vi "DB Read Queries.vi"(5 "Query info":T2, 7 "Query Command":T1, 8 "에러 입력(에러 없음)":errorcluster, 11 "참조 번호 입력":T3) -> (0 "에러 출력":errorcluster, 1 "Data (0번행)":string[](array[string]), 2 "Data":string[][](array[string]), 3 "참조 번호 출력":T3, 4 "None?":bool)   [LabVIEW 2020]
uses:
  <vilib>/addons/database/Connection.llb/Conn ObjectReference.ctl
  Controls/Clst_Query Info.ctl
  Controls/Cmd_Read Query.ctl
  Variables/Global_Cal Info.vi
  <vilib>/addons/database/NI_Database_API.lvlib
panel:
  out "Query":string
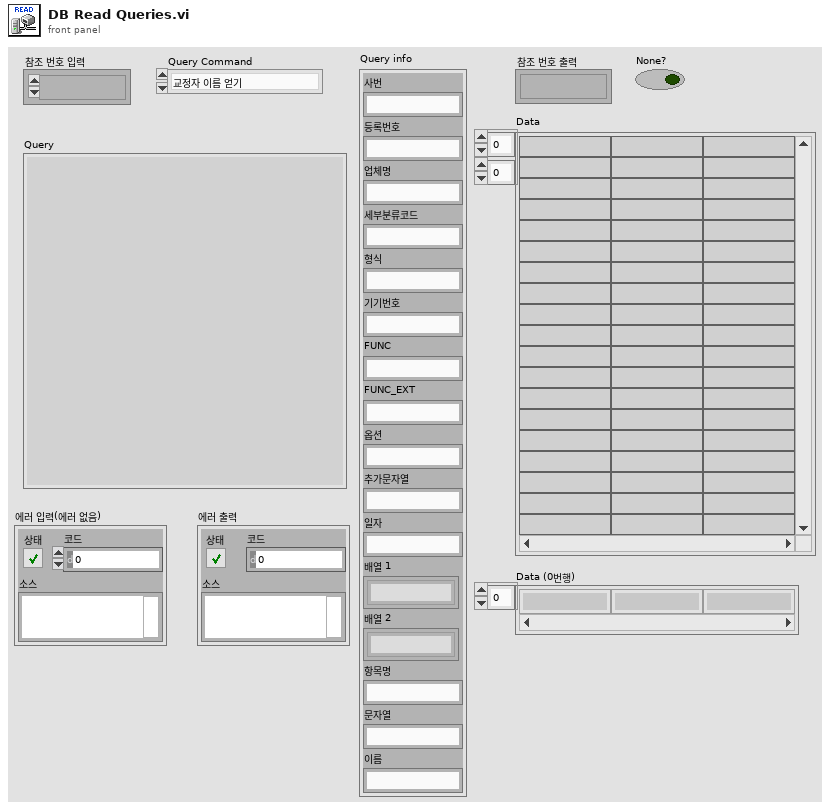
[diagram p1: front panel]
types:
  T1 = typedef "Cmd_Read Query.ctl" = enum16{"교정자 이름 얻기", "인증교정자 얻기", "기술책임자 얻기", "기책부책 얻기", "등록번호 얻기", "등록정보 얻기", "업체정보 얻기", "교정일자(CAMAS) 얻기", "교정일자(CALSTD) 얻기", "교정환경 얻기", "교정절차서 목록 얻기", "교정절차서명 얻기", "교정절차 목록얻기", "교정절차 얻기", "PROC 교정절차 얻기", "PROC SPEC 얻기", "교정절차(Func별) 얻기", "교정절차(Func_ext별) 얻기", "기관코드 얻기", "교정기능(세부분류) 얻기", "교정기능(모델) 얻기", "교정기능 목록 얻기", "교정기능 명칭 얻기", "교정기능 항목명칭 얻기", "DB (사용기준기) 얻기", "DB (기준기이름) 얻기", "DB (기준기이름목록) 얻기", "DB (기준기목록) 얻기", "DB (기준기값) 얻기", "DB (CMC) 얻기", "DB (FUNC) 얻기", "DB (CALNAME) 얻기", "DB (STDNAME) 얻기", "DB (SPEC) 얻기", "모델(항목전체) 얻기", "모델(최대범위) 얻기", "모델(최소범위) 얻기", "모델(최대최소) 얻기", "모델(범위조건) 얻기", "모델(등록요청) 얻기", "모델(형식별) 얻기", "모델(조건별) 얻기", "모델(모델검색) 얻기", "세부분류 목록 얻기", "기준기등록리스트 얻기", "STD Cal Date Check", "DB등록일자 얻기", "적용항목 얻기", "기타정보 얻기", "기준기요청 얻기", "서버버전 얻기"}
  T2 = typedef "Clst_Query Info.ctl" = cluster{"사번":string, "등록번호":string, "업체명":string, "세부분류코드":string, "형식":string, "기기번호":string, "FUNC":string, "FUNC_EXT":string, "옵션":string, "추가문자열":string, "일자":string, "배열 1":string[], "배열 2":string[], "항목명":string, "문자열":string, "이름":string}
  T3 = typedef "NI_Database_API.lvlib/Conn ObjectReference.ctl" = refnum<k1>
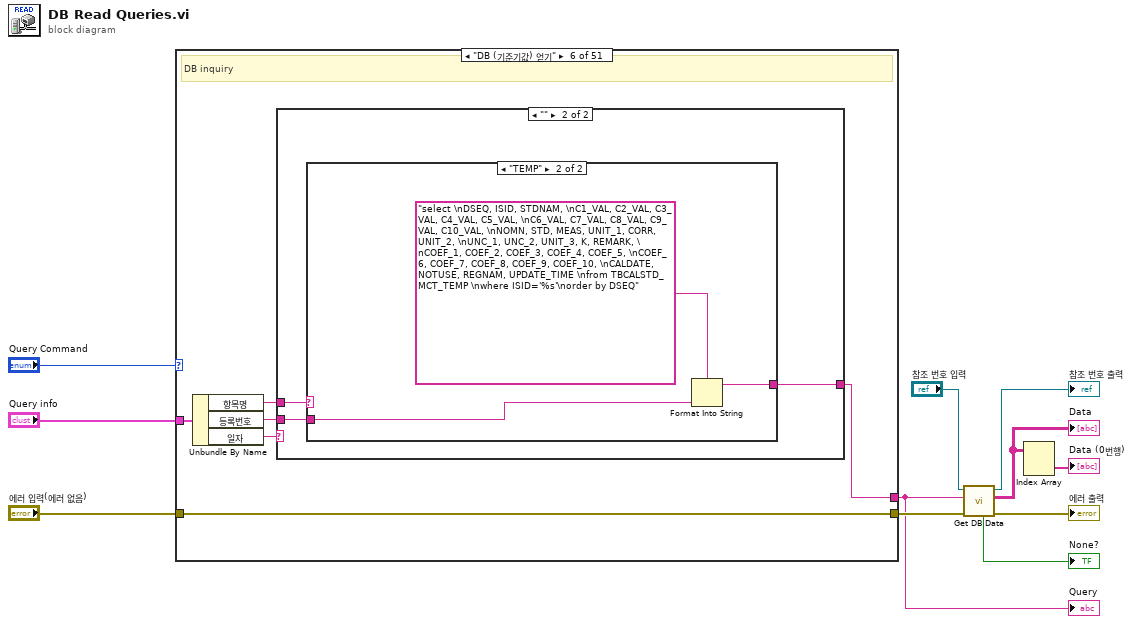
[diagram p0: block diagram]
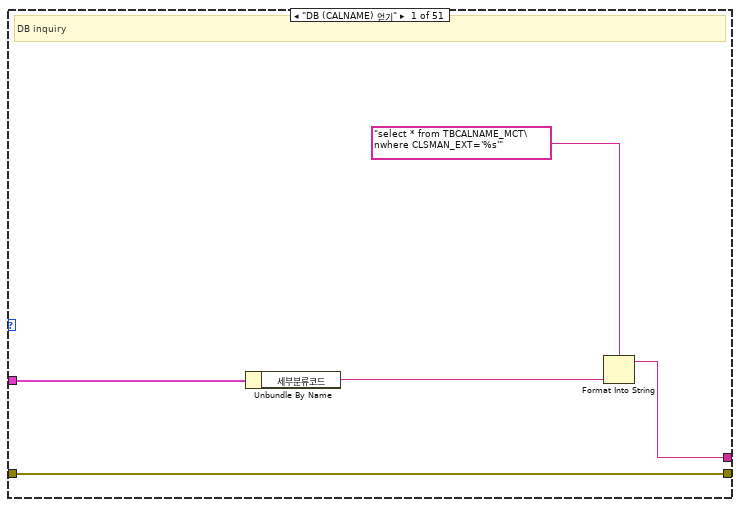
[diagram p2: hidden frame]
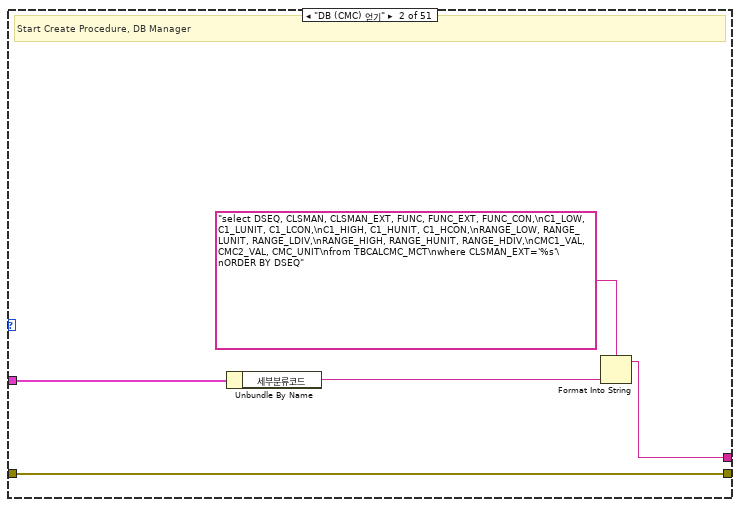
[diagram p3: hidden frame]
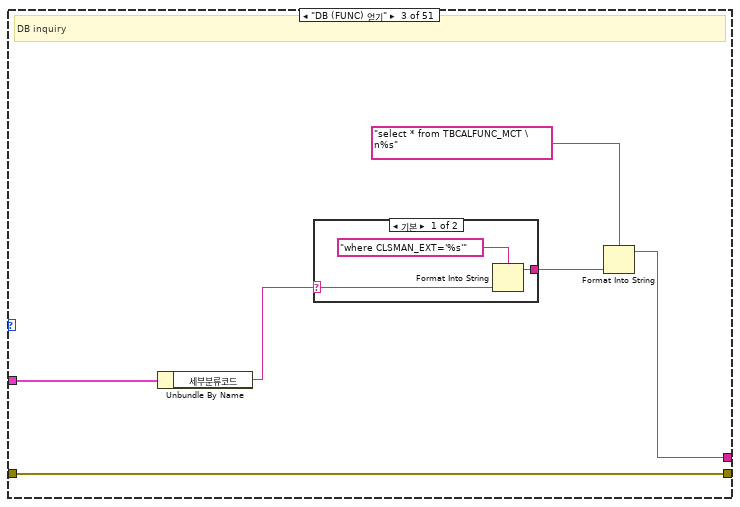
[diagram p4: hidden frame]
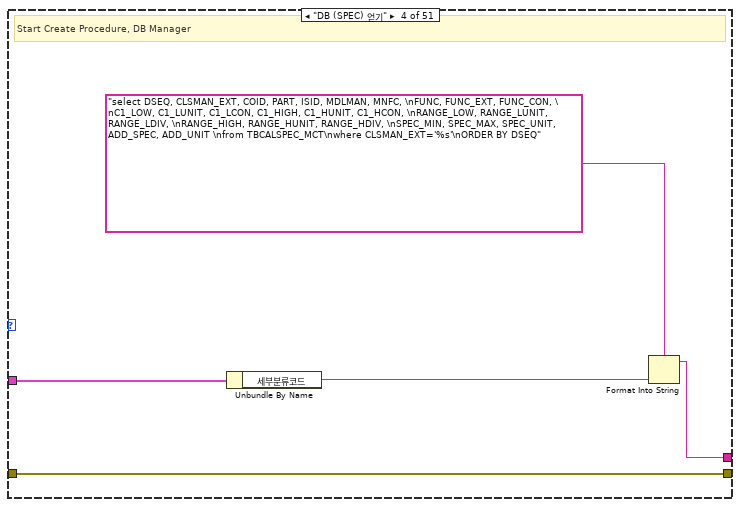
[diagram p6: hidden frame]
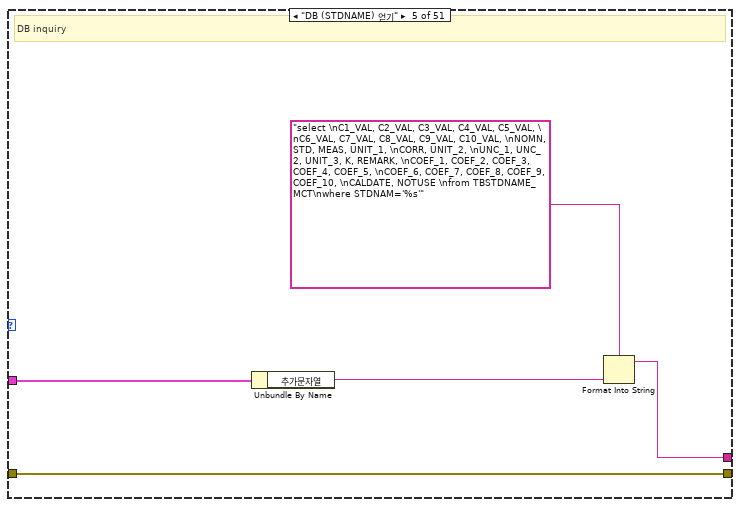
[diagram p7: hidden frame]
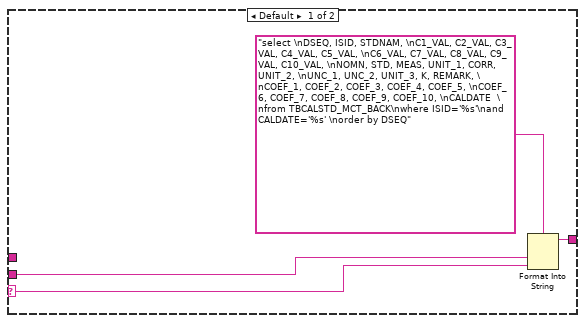
[diagram p8: hidden frame]
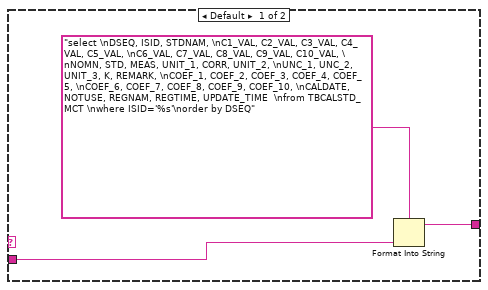
[diagram p9: hidden frame]
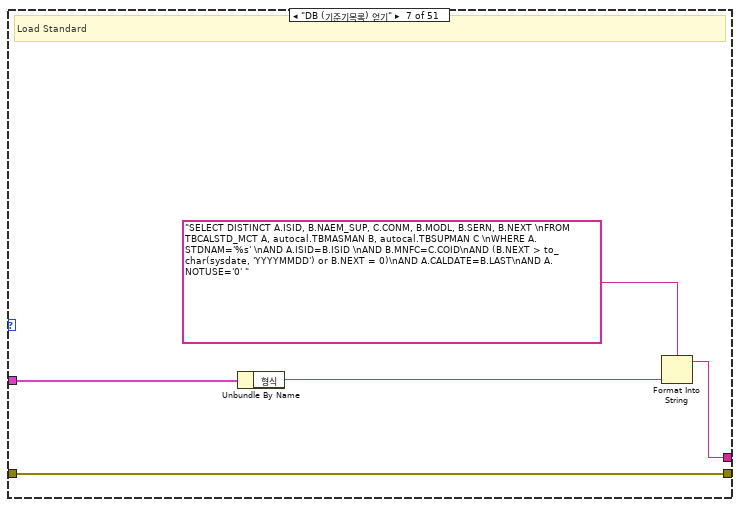
[diagram p10: hidden frame]
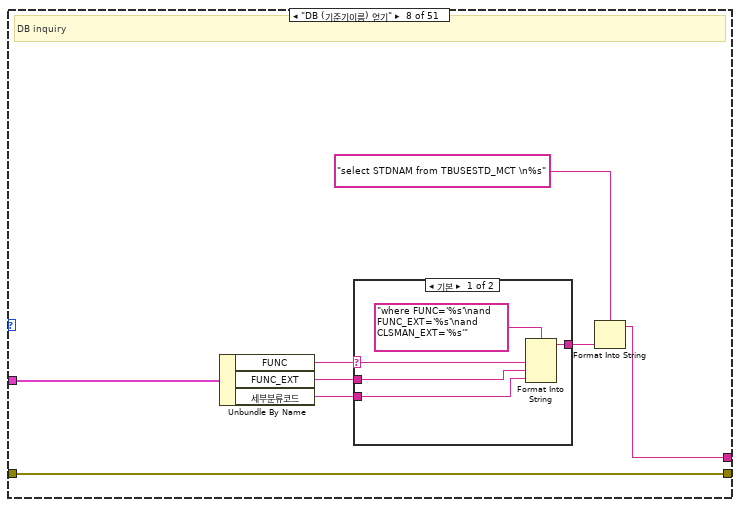
[diagram p11: hidden frame]
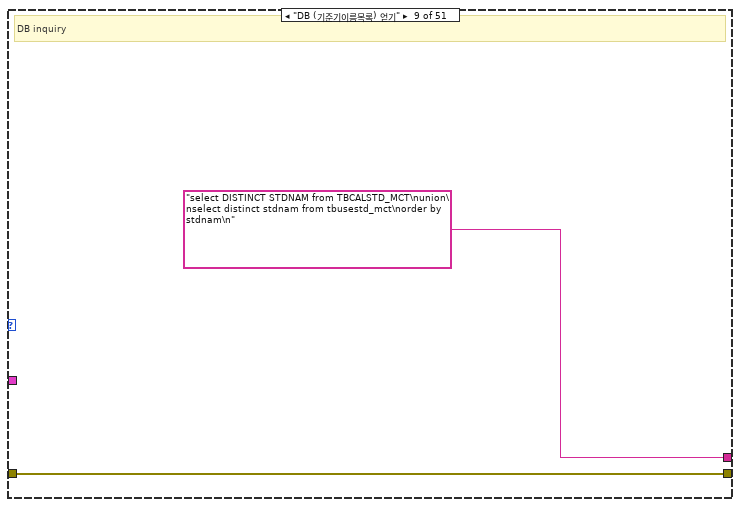
[diagram p13: hidden frame]
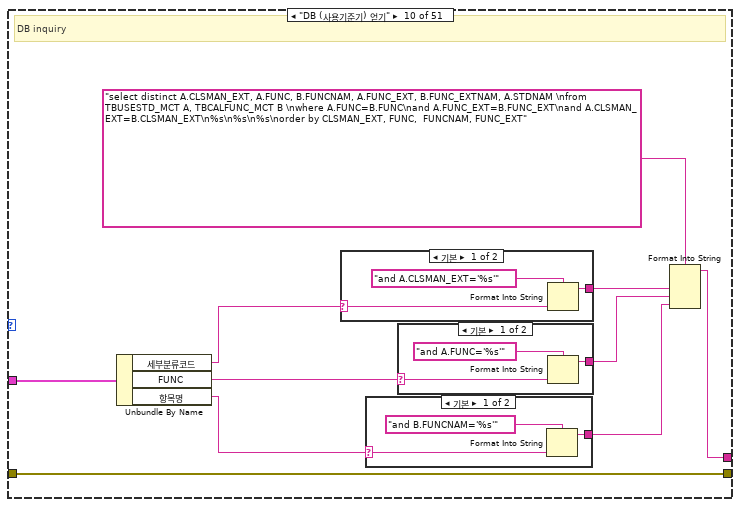
[diagram p14: hidden frame]
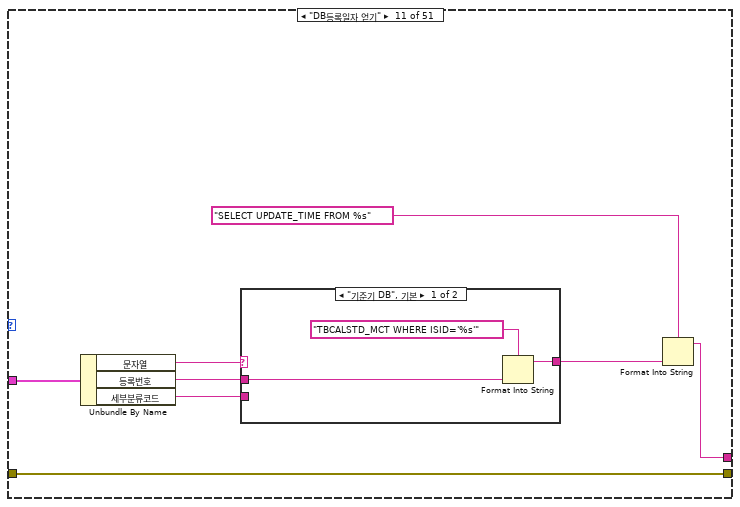
[diagram p18: hidden frame]
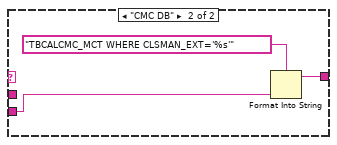
[diagram p19: hidden frame]
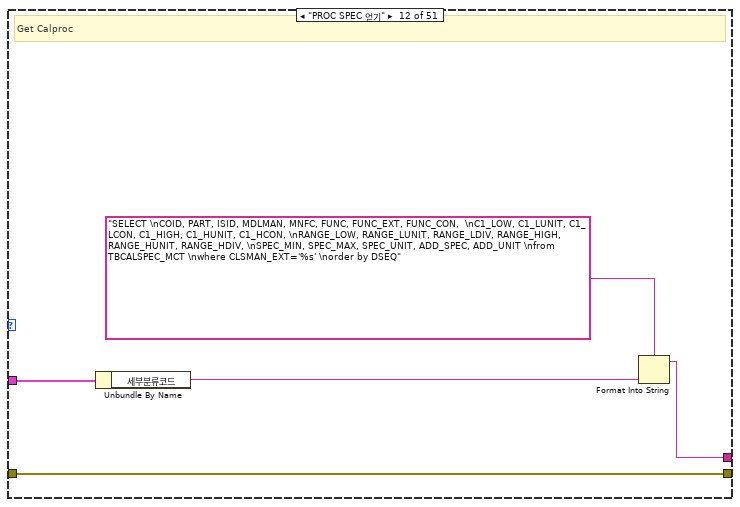
[diagram p20: hidden frame]
diagram:
  n1 = case shown="\"DB (기준기값) 얻기\"" "Query Command" {
    tunnel: "에러 입력(에러 없음)" -> [w16 w21 w27 w35 w40 w46 w64 w72 w79 w89 w106 w117 w127 w138 w155 w160 w165 w175 w186 w191 w196 w201 w209 w229 w248 w267 w278 w283 w304 w327 w332 w357 w365 w371 w376 w377 w386 w388 w397 w414 w431 w442 w457 w464 w476 w484 w490 w492 w497 w507 w521]
    tunnel: [w16 w21 w27 w35 w40 w46 w64 w72 w79 w89 w106 w117 w127 w138 w155 w160 w165 w175 w186 w191 w196 w201 w209 w229 w248 w267 w278 w283 w304 w327 w332 w357 w365 w371 w376 w377 w386 w388 w397 w414 w431 w442 w457 w464 w476 w484 w490 w492 w497 w507 w521] -> w6
    tunnel: "Query info" -> [w14 w20 w26 w34 w38 w45 w62 w71 _ w88 w105 w114 w118 w135 w154 _ w164 w174 w185 w190 w194 w197 w208 w226 w245 w264 w277 w282 w294 w326 w335 w353 w363 _ w375 w380 w384 _ w392 w413 w428 w441 w456 w463 w475 w483 _ _ w495 w506 _]
    tunnel: [w12 w17 w24 w31 w36 w42 w60 w69 "select DISTINCT STDNAM from TBCALSTD_MCT\nunion\nselect distinct stdnam from tbusestd_mct\norder by stdnam\n" w86 w103 w113 w123 w136 w152 "select CLSMAN_EXT, FUNC, FUNCNAM, FUNC_EXT, FUNC_EXTNAM\nfrom TBCALFUNC_MCT\norder by clsman_ext" ("포맷 문자열") w162 w172 w182 w188 w192 w200 w202 w228 w247 w266 w274 w279 w303 w323 w333 w354 w364 "select distinct emid from autocal.tbcetman\nwhere clas='기술책임자(정)'\nor clas='기술책임자(부)'\norder by emid" ("SQL query") w373 w378 w382 "SELECT DISTINCT REGTYP, CLSMAN_EXT, EQPNAM, MDLMAN, OPT_CODE, REGNAM, \nSUBSTR(UPDATE_TIME,0, 10) \nFROM TBCALPROC_MCT_TEMP \nORDER BY CLSMAN_EXT, MDLMAN, OPT_CODE" w393 w410 w429 w440 w455 w462 w472 w481 "SELECT mct_ver, ftp_ver FROM TBMCTVERMAN" ("SQL query") "select distinct clsman_ext, coddes_ext\nfrom autocal.tbclsman\nwhere stdnam is not null\norder by clsman_ext" ("SQL query") w493 w502 "SELECT DISTINCT A.CLSMAN_EXT, B.CODDES_EXT\nFROM\nTBCALFUNC_MCT A, AUTOCAL.TBCLSMAN B\nWHERE A.CLSMAN_EXT=B.CLSMAN_EXT\nORDER BY A.CLSMAN_EXT"] -> w3
    frame "DB (CALNAME) 얻기" {
      # "DB inquiry"
      n2 = Unbundle By Name(w14) -> ("세부분류코드"=w15:string)
      n3 = Format Into String(format string="select * from TBCALNAME_MCT\nwhere CLSMAN_EXT='%s'", w15) -> (resulting string=w12:string)  [unwired: 2 in, 1 out]
    }
    frame "DB (CMC) 얻기" {
      # "Start Create Procedure, DB Manager"
      n4 = Unbundle By Name(w20) -> ("세부분류코드"=w18:string)
      n5 = Format Into String(format string="select DSEQ, CLSMAN, CLSMAN_EXT, FUNC, FUNC_EXT, FUNC_CON,\nC1_LOW, C1_LUNIT, C1_LCON,\nC1_HIGH, C1_HUNIT, C1_HCON,\nRANGE_LOW, RANGE_LUNIT, RANGE_LDIV,\nRANGE_HIGH, RANGE_HUNIT, RANGE_HDIV,\nCMC1_VAL, CMC2_VAL, CMC_UNIT\nfrom TBCALCMC_MCT\nwhere CLSMAN_EXT='%s'\nORDER BY DSEQ", w18) -> (resulting string=w17:string)  [unwired: 2 in, 1 out]
    }
    frame "DB (FUNC) 얻기" {
      # "DB inquiry"
      n6 = Unbundle By Name(w26) -> ("세부분류코드"=w23:string)
      n7 = case shown="기본" w23 {
        selector: w23 -> [w30 _]
        tunnel: [w29 _] -> w22
        frame Default {
          n8 = Format Into String(format string="where CLSMAN_EXT='%s'", w30) -> (resulting string=w29:string)  [unwired: 2 in, 1 out]
        }
        frame "" {
        }
      }
      n9 = Format Into String(format string="select * from TBCALFUNC_MCT \n%s", w22) -> (resulting string=w24:string)  [unwired: 2 in, 1 out]
    }
    frame "DB (SPEC) 얻기" {
      # "Start Create Procedure, DB Manager"
      n10 = Unbundle By Name(w34) -> ("세부분류코드"=w32:string)
      n11 = Format Into String(format string="select DSEQ, CLSMAN_EXT, COID, PART, ISID, MDLMAN, MNFC, \nFUNC, FUNC_EXT, FUNC_CON, \nC1_LOW, C1_LUNIT, C1_LCON, C1_HIGH, C1_HUNIT, C1_HCON, \nRANGE_LOW, RANGE_LUNIT, RANGE_LDIV, \nRANGE_HIGH, RANGE_HUNIT, RANGE_HDIV, \nSPEC_MIN, SPEC_MAX, SPEC_UNIT, ADD_SPEC, ADD_UNIT \nfrom TBCALSPEC_MCT\nwhere CLSMAN_EXT='%s'\nORDER BY DSEQ", w32) -> (resulting string=w31:string)  [unwired: 2 in, 1 out]
    }
    frame "DB (STDNAME) 얻기" {
      # "DB inquiry"
      n12 = Unbundle By Name(w38) -> ("추가문자열"=w39:string)
      n13 = Format Into String(format string="select \nC1_VAL, C2_VAL, C3_VAL, C4_VAL, C5_VAL, \nC6_VAL, C7_VAL, C8_VAL, C9_VAL, C10_VAL, \nNOMN, STD, MEAS, UNIT_1, \nCORR, UNIT_2, \nUNC_1, UNC_2, UNIT_3, K, REMARK, \nCOEF_1, COEF_2, COEF_3, COEF_4, COEF_5, \nCOEF_6, COEF_7, COEF_8, COEF_9, COEF_10, \nCALDATE, NOTUSE \nfrom TBSTDNAME_MCT\nwhere STDNAM='%s'", w39) -> (resulting string=w36:string)  [unwired: 2 in, 1 out]
    }
    frame "DB (기준기값) 얻기" {
      # "DB inquiry"
      n14 = Unbundle By Name(w45) -> ("항목명"=w41:string, "등록번호"=w43:string, "일자"=w44:string)
      n15 = case shown="\"\"" w44 {
        selector: w44 -> [w50 _]
        tunnel: w43 -> [w49 w53]
        tunnel: [w47 w52] -> w42
        tunnel: w41 -> [_ w51]
        frame Default {
          n16 = Format Into String(format string="select \nDSEQ, ISID, STDNAM, \nC1_VAL, C2_VAL, C3_VAL, C4_VAL, C5_VAL, \nC6_VAL, C7_VAL, C8_VAL, C9_VAL, C10_VAL, \nNOMN, STD, MEAS, UNIT_1, CORR, UNIT_2, \nUNC_1, UNC_2, UNIT_3, K, REMARK, \nCOEF_1, COEF_2, COEF_3, COEF_4, COEF_5, \nCOEF_6, COEF_7, COEF_8, COEF_9, COEF_10, \nCALDATE  \nfrom TBCALSTD_MCT_BACK\nwhere ISID='%s'\nand CALDATE='%s' \norder by DSEQ", w49, w50) -> (resulting string=w47:string)  [unwired: 2 in, 1 out]
        }
        frame "" {
          n17 = case shown="\"TEMP\"" w51 {
            tunnel: w53 -> [w55 w58]
            tunnel: [w54 w57] -> w52
            frame Default {
              n18 = Format Into String(format string="select \nDSEQ, ISID, STDNAM, \nC1_VAL, C2_VAL, C3_VAL, C4_VAL, C5_VAL, \nC6_VAL, C7_VAL, C8_VAL, C9_VAL, C10_VAL, \nNOMN, STD, MEAS, UNIT_1, CORR, UNIT_2, \nUNC_1, UNC_2, UNIT_3, K, REMARK, \nCOEF_1, COEF_2, COEF_3, COEF_4, COEF_5, \nCOEF_6, COEF_7, COEF_8, COEF_9, COEF_10, \nCALDATE, NOTUSE, REGNAM, REGTIME, UPDATE_TIME  \nfrom TBCALSTD_MCT \nwhere ISID='%s'\norder by DSEQ", w55) -> (resulting string=w54:string)  [unwired: 2 in, 1 out]
            }
            frame "TEMP" {
              n19 = Format Into String(format string="select \nDSEQ, ISID, STDNAM, \nC1_VAL, C2_VAL, C3_VAL, C4_VAL, C5_VAL, \nC6_VAL, C7_VAL, C8_VAL, C9_VAL, C10_VAL, \nNOMN, STD, MEAS, UNIT_1, CORR, UNIT_2, \nUNC_1, UNC_2, UNIT_3, K, REMARK, \nCOEF_1, COEF_2, COEF_3, COEF_4, COEF_5, \nCOEF_6, COEF_7, COEF_8, COEF_9, COEF_10, \nCALDATE, NOTUSE, REGNAM, UPDATE_TIME \nfrom TBCALSTD_MCT_TEMP \nwhere ISID='%s'\norder by DSEQ", w58) -> (resulting string=w57:string)  [unwired: 2 in, 1 out]
            }
          }
        }
      }
    }
    frame "DB (기준기목록) 얻기" {
      # "Load Standard"
      n20 = Unbundle By Name(w62) -> ("형식"=w61:string)
      n21 = Format Into String(format string="SELECT DISTINCT A.ISID, B.NAEM_SUP, C.CONM, B.MODL, B.SERN, B.NEXT \nFROM TBCALSTD_MCT A, autocal.TBMASMAN B, autocal.TBSUPMAN C \nWHERE A.STDNAM='%s' \nAND A.ISID=B.ISID \nAND B.MNFC=C.COID\nAND (B.NEXT > to_char(sysdate, 'YYYYMMDD') or B.NEXT = 0)\nAND A.CALDATE=B.LAST\nAND A.NOTUSE='0' ", w61) -> (resulting string=w60:string)  [unwired: 2 in, 1 out]
    }
    frame "DB (기준기이름) 얻기" {
      # "DB inquiry"
      n22 = Unbundle By Name(w71) -> ("FUNC"=w66:string, "FUNC_EXT"=w68:string, "세부분류코드"=w65:string)
      n23 = case shown="기본" w66 {
        selector: w66 -> [w74 _]
        tunnel: w68 -> [w76 _]
        tunnel: [w75 _] -> w67
        tunnel: w65 -> [w73 _]
        frame Default {
          n24 = Format Into String(format string="where FUNC='%s'\nand FUNC_EXT='%s'\nand CLSMAN_EXT='%s'" ("포맷 문자열"), w74, w76, w73) -> (resulting string=w75:string)  [unwired: 2 in, 1 out]
        }
        frame "" {
        }
      }
      n25 = Format Into String(format string="select STDNAM from TBUSESTD_MCT \n%s", w67) -> (resulting string=w69:string)  [unwired: 2 in, 1 out]
    }
    frame "DB (기준기이름목록) 얻기" {
      # "DB inquiry"
    }
    frame "DB (사용기준기) 얻기" {
      # "DB inquiry"
      n26 = Unbundle By Name(w88) -> ("세부분류코드"=w81:string, "FUNC"=w85:string, "항목명"=w83:string)
      n27 = case shown="기본" w81 {
        selector: w81 -> [w92 _]
        tunnel: [w91 _] -> w80
        frame Default {
          n28 = Format Into String(format string="and A.CLSMAN_EXT='%s'" ("포맷 문자열"), w92) -> (resulting string=w91:string)  [unwired: 2 in, 1 out]
        }
        frame "" {
        }
      }
      n29 = case shown="기본" w83 {
        selector: w83 -> [w95 _]
        tunnel: [w94 _] -> w82
        frame Default {
          n30 = Format Into String(format string="and B.FUNCNAM='%s'" ("포맷 문자열"), w95) -> (resulting string=w94:string)  [unwired: 2 in, 1 out]
        }
        frame "" {
        }
      }
      n31 = case shown="기본" w85 {
        selector: w85 -> [w98 _]
        tunnel: [w97 _] -> w84
        frame Default {
          n32 = Format Into String(format string="and A.FUNC='%s'" ("포맷 문자열"), w98) -> (resulting string=w97:string)  [unwired: 2 in, 1 out]
        }
        frame "" {
        }
      }
      n33 = Format Into String(format string="select distinct A.CLSMAN_EXT, A.FUNC, B.FUNCNAM, A.FUNC_EXT, B.FUNC_EXTNAM, A.STDNAM \nfrom TBUSESTD_MCT A, TBCALFUNC_MCT B \nwhere A.FUNC=B.FUNC\nand A.FUNC_EXT=B.FUNC_EXT\nand A.CLSMAN_EXT=B.CLSMAN_EXT\n%s\n%s\n%s\norder by CLSMAN_EXT, FUNC,  FUNCNAM, FUNC_EXT", w80, w84, w82) -> (resulting string=w86:string)  [unwired: 2 in, 1 out]
    }
    frame "DB등록일자 얻기" {
      n34 = Unbundle By Name(w105) -> ("문자열"=w102:string, "등록번호"=w100:string, "세부분류코드"=w99:string)
      n35 = case shown="\"기준기 DB\", 기본" w102 {
        tunnel: [w107 w111] -> w101
        tunnel: w100 -> [w108 _]
        tunnel: w99 -> [_ w110]
        frame "기준기 DB", Default {
          n36 = Format Into String(format string="TBCALSTD_MCT WHERE ISID='%s'" ("포맷 문자열"), w108) -> (resulting string=w107:string)  [unwired: 2 in, 1 out]
        }
        frame "CMC DB" {
          n37 = Format Into String(format string="TBCALCMC_MCT WHERE CLSMAN_EXT='%s'" ("포맷 문자열"), w110) -> (resulting string=w111:string)  [unwired: 2 in, 1 out]
        }
      }
      n38 = Format Into String(format string="SELECT UPDATE_TIME FROM %s", w101) -> (resulting string=w103:string)  [unwired: 2 in, 1 out]
    }
    frame "PROC SPEC 얻기" {
      # "Get Calproc"
      n39 = Unbundle By Name(w114) -> ("세부분류코드"=w116:string)
      n40 = Format Into String(format string="SELECT \nCOID, PART, ISID, MDLMAN, MNFC, FUNC, FUNC_EXT, FUNC_CON,  \nC1_LOW, C1_LUNIT, C1_LCON, C1_HIGH, C1_HUNIT, C1_HCON, \nRANGE_LOW, RANGE_LUNIT, RANGE_LDIV, RANGE_HIGH, RANGE_HUNIT, RANGE_HDIV, \nSPEC_MIN, SPEC_MAX, SPEC_UNIT, ADD_SPEC, ADD_UNIT \nfrom TBCALSPEC_MCT \nwhere CLSMAN_EXT='%s' \norder by DSEQ", w116) -> (resulting string=w113:string)  [unwired: 2 in, 1 out]
    }
    frame "PROC 교정절차 얻기" {
      # "Get Calproc"
      n41 = Unbundle By Name(w118) -> ("추가문자열"=w122:string, "세부분류코드"=w125:string, "형식"=w126:string, "옵션"=w120:string)
      n42 = case shown="기본" w122 {
        tunnel: ["TBCALPROC_MCT" ("추가문자열") "TBCALPROC_MCT_TEMP" ("추가문자열")] -> w121
        frame Default {
        }
        frame "TEMP" {
        }
      }
      n43 = case shown="기본" w120 {
        selector: w120 -> [w129 _]
        tunnel: [w128 "AND OPT_CODE is null"] -> w119
        frame Default {
          n44 = Format Into String(format string="AND OPT_CODE='%s'", w129) -> (resulting string=w128:string)  [unwired: 2 in, 1 out]
        }
        frame "" {
        }
      }
      n45 = Format Into String(format string="SELECT\nDSEQ, FUNC, FUNC_EXT, \nCAL_VAL, CAL_UNIT, DISP_SYS, RESOL, RESOL_UNIT, \nC1_VAL, C2_VAL, C3_VAL, C4_VAL, C5_VAL,\nC6_VAL, C7_VAL, C8_VAL, C9_VAL, C10_VAL\nFROM %s\nWHERE CLSMAN_EXT='%s'\nAND MDLMAN='%s'\n%s\norder by DSEQ", w121, w125, w126, w119) -> (resulting string=w123:string)  [unwired: 2 in, 1 out]
    }
    frame "STD Cal Date Check" {
      n46 = Unbundle By Name(w135) -> ("옵션"=w134:string)
      n47 = case shown="\"2\"" w134 {
        tunnel: "select DISTINCT\nA.isid, B.naem_sup, TRIM(C.conm),\nB.modl, B.last, A.caldate, B.next,\nD.desn, E.desn\nfrom\nTBCALSTD_MCT A,\nautocal.TBMASMAN B,\nautocal.TBSUPMAN C,\nautocal.TBSTAMAN D, \nautocal.TBTYPMAN E\nwhere A.isid=B.isid \nAND B.mnfc=C.coid\nAND B.stat=D.stat\nAND B.tyep=E.tyep\nAND A.notuse='0'\n%s\norder by naem_sup" ("SQL query") -> [w139 w147]
        tunnel: [w140 w142] -> w136
        frame "1", Default {
          n48 = Format Into String(format string=w139, "AND A.caldate<>B.last" ("SQL query")) -> (resulting string=w140:string)  [unwired: 2 in, 1 out]
        }
        frame "2" {
          n49 = Format Date/Time String(time format string (%c)="%Y%m%d" ("시간 포맷 문자열 (%c)")) -> (date/time string=w145:string)  [unwired: 2 in]
          n50 = Format Into String(format string="AND B.next<'%s'\nAND B.next<>'0'" ("SQL query"), w145) -> (resulting string=w146:string)  [unwired: 2 in, 1 out]
          n51 = Format Into String(format string=w147, w146) -> (resulting string=w142:string)  [unwired: 2 in, 1 out]
        }
      }
    }
    frame "교정기능 명칭 얻기" {
      # "Get Cal Func List"
      n52 = Unbundle By Name(w154) -> ("FUNC"=w149:string, "세부분류코드"=w148:string, "FUNC_EXT"=w151:string)
      n53 = case shown="기본" w151 {
        selector: w151 -> [w157 _]
        tunnel: [w156 _] -> w150
        frame Default {
          n54 = Format Into String(format string="AND FUNC_EXT='%s'", w157) -> (resulting string=w156:string)  [unwired: 2 in, 1 out]
        }
        frame "" {
        }
      }
      n55 = Format Into String(format string="SELECT distinct func, funcnam, func_ext, func_extnam \nFROM TBCALFUNC_MCT \nWHERE FUNC='%s'\n%s\nAND CLSMAN_EXT='%s'", w149, w150, w148) -> (resulting string=w152:string)  [unwired: 2 in, 1 out]
    }
    frame "교정기능 목록 얻기" {
    }
    frame "교정기능 항목명칭 얻기" {
      # "DB Manager"
      n56 = Unbundle By Name(w164) -> ("세부분류코드"=w163:string)
      n57 = Format Into String(format string="select \nfunc, func_ext, \nc1_name, c2_name, c3_name, c4_name, c5_name, \nc6_name, c7_name, c8_name, c9_name, c10_name, \ncal_name, cal_unit, disp_sys, resol, resol_unit\nfrom TBCALNAME_MCT \nwhere \nCLSMAN_EXT='%s'" ("포맷 문자열"), w163) -> (resulting string=w162:string)  [unwired: 2 in, 1 out]
    }
    frame "교정기능(모델) 얻기" {
      # "Get Cal Func"
      n58 = Unbundle By Name(w174) -> ("추가문자열"=w168:string, "세부분류코드"=w173:string, "형식"=w170:string, "옵션"=w167:string)
      n59 = case shown="기본" w168 {
        tunnel: ["TBCALPROC_MCT" ("추가문자열") "TBCALPROC_MCT_TEMP" ("추가문자열")] -> w169
        frame Default {
        }
        frame "TEMP" {
        }
      }
      n60 = case shown="기본" w167 {
        selector: w167 -> [w177 _]
        tunnel: [w176 "AND OPT_CODE is null"] -> w166
        frame Default {
          n61 = Format Into String(format string="AND OPT_CODE='%s'", w177) -> (resulting string=w176:string)  [unwired: 2 in, 1 out]
        }
        frame "" {
        }
      }
      n62 = Format Into String(format string="select dseq, func, func_ext \nfrom %s\nwhere clsman_ext='%s' \nand mdlman='%s'\n%s\nORDER BY dseq", w169, w173, w170, w166) -> (resulting string=w172:string)  [unwired: 2 in, 1 out]
    }
    frame "교정기능(세부분류) 얻기" {
      # "Start Create Procedure"
      n63 = Unbundle By Name(w185) -> ("세부분류코드"=w183:string)
      n64 = Format Into String(format string="select A.func, A.funcnam, A.func_ext, A.func_extnam, B.coddes_ext\nfrom TBCALFUNC_MCT A, autocal.tbclsman B\nwhere A.clsman_ext='%s'\nAND A.clsman_ext=B.clsman_ext\norder by func_ext", w183) -> (resulting string=w182:string)  [unwired: 2 in, 1 out]
    }
    frame "교정일자(CALSTD) 얻기" {
      # "DB Manager"
      n65 = Unbundle By Name(w190) -> ("등록번호"=w189:string)
      n66 = Format Into String(format string="select distinct CALDATE \nfrom TBCALSTD_MCT_BACK \nwhere ISID='%s'\norder by CALDATE" ("SQL query"), w189) -> (resulting string=w188:string)  [unwired: 2 in, 1 out]
    }
    frame "교정일자(CAMAS) 얻기" {
      # "DB Manager"
      n67 = Unbundle By Name(w194) -> ("등록번호"=w193:string)
      n68 = Format Into String(format string="select LAST \nfrom autocal.tbmasman \nwhere ISID='%s'" ("SQL query"), w193) -> (resulting string=w192:string)  [unwired: 2 in, 1 out]
    }
    frame "교정자 이름 얻기", Default {
      # "Main, Get Basic Info"
      n69 = Unbundle By Name(w197) -> ("사번"=w198:string)
      n70 = Format Into String(format string="select emnm \nfrom autocal.tbempman \nwhere emid='%s' " ("포맷 문자열"), w198) -> (resulting string=w200:string)  [unwired: 2 in, 1 out]
    }
    frame "교정절차 목록얻기" {
      # "Get Cal Proc List"
      n71 = Unbundle By Name(w208) -> ("추가문자열"=w207:string, "세부분류코드"=w204:string, "형식"=w203:string)
      n72 = To Upper Case(1:w207) -> (0:w206:string)
      n73 = call <vilib>:"Trim Whitespace.vi"("string"=w206) -> ("trimmed string"=w205:string)  [unwired: 1 in]
      n74 = case shown="기본" w205 {
        tunnel: [w212 w216] -> w202
        tunnel: w204 -> [w210 w215]
        tunnel: w203 -> [w211 w214]
        frame Default {
          n75 = Format Into String(format string="select DISTINCT\nclsman, clsman_ext, eqpnam, mdlman, opt_code, c1_val\nfrom TBCALPROC_MCT\nwhere CLSMAN_EXT='%s'\nAND MDLMAN='설정'\nUNION\nselect DISTINCT\nclsman, clsman_ext, eqpnam, mdlman, opt_code, c1_val \nfrom TBCALPROC_MCT\nwhere CLSMAN_EXT='%s' \nAND MDLMAN='%s' \nUNION\nselect DISTINCT\nclsman, clsman_ext, eqpnam, mdlman, opt_code, c1_val \nfrom TBCALPROC_MCT\nwhere CLSMAN_EXT='%s' \nAND MDLMAN='ALL' \n\norder by mdlman, opt_code", w210, w210, w211, w210) -> (resulting string=w212:string)  [unwired: 2 in, 1 out]
        }
        frame "TEMP" {
          n76 = Format Into String(format string="select DISTINCT\nclsman, clsman_ext, eqpnam, mdlman, opt_code, c1_val \nfrom TBCALPROC_MCT_TEMP\nwhere CLSMAN_EXT='%s' \nAND MDLMAN='%s' \norder by mdlman, opt_code", w215, w214) -> (resulting string=w216:string)  [unwired: 2 in, 1 out]
        }
      }
    }
    frame "교정절차 얻기" {
      # "Insert proc_temp, DB Manager, DB inquiry"
      n77 = Unbundle By Name(w226) -> ("추가문자열"=w223:string, "세부분류코드"=w225:string, "형식"=w224:string, "옵션"=w219:string)
      n78 = To Upper Case(1:w223) -> (0:w222:string)
      n79 = call <vilib>:"Trim Whitespace.vi"("string"=w222) -> ("trimmed string"=w221:string)  [unwired: 1 in]
      n80 = case shown="기본" w219 {
        selector: w219 -> [w231 _]
        tunnel: [w230 "AND OPT_CODE is null"] -> w218
        frame Default {
          n81 = Format Into String(format string="AND OPT_CODE='%s'", w231) -> (resulting string=w230:string)  [unwired: 2 in, 1 out]
        }
        frame "" {
        }
      }
      n82 = case shown="기본" w221 {
        tunnel: ["TBCALPROC_MCT" ("추가문자열") "TBCALPROC_MCT_TEMP" ("추가문자열")] -> w220
        frame Default {
        }
        frame "TEMP" {
        }
      }
      n83 = Format Into String(format string="select \nDSEQ, CLSMAN, CLSMAN_EXT, EQPNAM, \nMDLMAN, OPT_CODE, FUNC, FUNC_EXT, \nC1_VAL, C2_VAL, C3_VAL, C4_VAL, C5_VAL, \nC6_VAL, C7_VAL, C8_VAL, C9_VAL, C10_VAL,\nCAL_VAL, CAL_UNIT, DISP_SYS, RESOL, RESOL_UNIT, \nREGNAM, UPDATE_TIME \nfrom %s\nwhere CLSMAN_EXT='%s' \nAND MDLMAN='%s'\n%s\norder by DSEQ", w220, w225, w224, w218) -> (resulting string=w228:string)  [unwired: 2 in, 1 out]
    }
    frame "교정절차(Func_ext별) 얻기" {
      # "Insert proc_temp, DB Manager, DB inquiry"
      n84 = Unbundle By Name(w245) -> ("추가문자열"=w242:string, "세부분류코드"=w244:string, "형식"=w243:string, "옵션"=w237:string, "FUNC"=w240:string)
      n85 = To Upper Case(1:w242) -> (0:w241:string)
      n86 = call <vilib>:"Trim Whitespace.vi"("string"=w241) -> ("trimmed string"=w239:string)  [unwired: 1 in]
      n87 = case shown="\"\"" w237 {
        selector: w237 -> [w250 _]
        tunnel: [w249 "AND OPT_CODE is null"] -> w236
        frame Default {
          n88 = Format Into String(format string="AND OPT_CODE='%s'", w250) -> (resulting string=w249:string)  [unwired: 2 in, 1 out]
        }
        frame "" {
        }
      }
      n89 = case shown="기본" w239 {
        tunnel: ["TBCALPROC_MCT" ("추가문자열") "TBCALPROC_MCT_TEMP" ("추가문자열")] -> w238
        frame Default {
        }
        frame "TEMP" {
        }
      }
      n90 = Format Into String(format string="select \nDSEQ, CLSMAN, CLSMAN_EXT, EQPNAM, \nMDLMAN, OPT_CODE, FUNC, FUNC_EXT,\nC1_VAL, C2_VAL, C3_VAL, C4_VAL, C5_VAL, \nC6_VAL, C7_VAL, C8_VAL, C9_VAL, C10_VAL,\nCAL_VAL, CAL_UNIT, DISP_SYS, RESOL, RESOL_UNIT\nfrom %s\nwhere CLSMAN_EXT='%s' \nAND MDLMAN='%s'\n%s\nAND FUNC_EXT='%s'\norder by DSEQ", w238, w244, w243, w236, w240) -> (resulting string=w247:string)  [unwired: 2 in, 1 out]
    }
    frame "교정절차(Func별) 얻기" {
      # "Insert proc_temp, DB Manager, DB inquiry"
      n91 = Unbundle By Name(w264) -> ("추가문자열"=w261:string, "세부분류코드"=w263:string, "형식"=w262:string, "옵션"=w256:string, "FUNC"=w259:string)
      n92 = To Upper Case(1:w261) -> (0:w260:string)
      n93 = call <vilib>:"Trim Whitespace.vi"("string"=w260) -> ("trimmed string"=w258:string)  [unwired: 1 in]
      n94 = case shown="\"\"" w256 {
        selector: w256 -> [w269 _]
        tunnel: [w268 "AND OPT_CODE is null"] -> w255
        frame Default {
          n95 = Format Into String(format string="AND OPT_CODE='%s'", w269) -> (resulting string=w268:string)  [unwired: 2 in, 1 out]
        }
        frame "" {
        }
      }
      n96 = case shown="기본" w258 {
        tunnel: ["TBCALPROC_MCT" ("추가문자열") "TBCALPROC_MCT_TEMP" ("추가문자열")] -> w257
        frame Default {
        }
        frame "TEMP" {
        }
      }
      n97 = Format Into String(format string="select \nDSEQ, CLSMAN, CLSMAN_EXT, EQPNAM, \nMDLMAN, OPT_CODE, FUNC, FUNC_EXT,\nC1_VAL, C2_VAL, C3_VAL, C4_VAL, C5_VAL, \nC6_VAL, C7_VAL, C8_VAL, C9_VAL, C10_VAL,\nCAL_VAL, CAL_UNIT, DISP_SYS, RESOL, RESOL_UNIT\nfrom %s\nwhere CLSMAN_EXT='%s' \nAND MDLMAN='%s'\n%s\nAND FUNC='%s'\norder by DSEQ", w257, w263, w262, w255, w259) -> (resulting string=w266:string)  [unwired: 2 in, 1 out]
    }
    frame "교정절차서 목록 얻기" {
      # "Get Cal Proc Docu List"
      n98 = Unbundle By Name(w277) -> ("사번"=w275:string)
      n99 = Format Into String(format string="select distinct A.stdnam, A.calstd, A.clsman \nfrom autocal.tbclsman A, autocal.tbcetman B \nwhere A.calcls=B.calcls \nand A.stdnam is not null \nand B.emid='%s' \nand B.clas='기술책임자(정)' \nand not (A.clsman='10615' or A.clsman='10622') \norder by A.clsman", w275) -> (resulting string=w274:string)  [unwired: 2 in, 1 out]
    }
    frame "교정절차서명 얻기" {
      # "Get Basic Info"
      n100 = Unbundle By Name(w282) -> ("세부분류코드"=w280:string)
      n101 = Format Into String(format string="select coddes, calstd \nfrom autocal.tbclsman \nwhere clsman_ext='%s'", w280) -> (resulting string=w279:string)  [unwired: 2 in, 1 out]
    }
    frame "교정환경 얻기" {
      # "Get Environment"
      n102 = Unbundle By Name(w294) -> ("세부분류코드"=w300:string, "일자"=w291:string)
      n103 = global read "Global_Cal Info.vi" "룸구분"() -> (w293:string[][])
      n104 = Delete From Array(array=w293, length=3 ("길이"), index (col)=0 ("비활성화된 인덱스 (열)")) -> (deleted portion=w285:string[][], array with subset deleted=w299:string[][])  [unwired: 1 in]
      n105 = call <vilib>:"Trim Whitespace.vi"("string"=w300) -> ("trimmed string"=w290:string)  [unwired: 1 in]
      n106 = String Subset(string=w290, length (rest)=3 ("길이(나머지)")) -> (substring=w302:string)  [unwired: 1 in]
      n107 = for {
        tunnel: w299 -> [w310] mode=indexing
        tunnel: w302 -> [w309]
        tunnel: [w307] -> w287 mode=indexing if=w305
        tunnel: [w306] -> w284 mode=indexing if=w305
        tunnel: w285 -> [w306] mode=indexing
        i -> [w307]
        n108 = Search 1D Array(1D array=w310, element=w309) -> (index of element=w308:i32)  [unwired: 1 in]
        n109 = Greater Or Equal To 0?(x=w308) -> (x >= 0?=w305:bool)
      }
      n110 = Array Size(array=w287) -> (size(s)=w289:i32)
      n111 = case shown="기본" w289 {
        tunnel: w287 -> [_ w313 w316]
        tunnel: [1 w312 w314] -> w286
        tunnel: w284 -> [_ _ w320]
        frame 0 {
        }
        frame 1 {
          n112 = Index Array(array=w313) -> (element=w312:i32)  [unwired: 1 in]
        }
        frame Default {
          n113 = call "User select_listbox.vi"("리스트명"="교정실선택", "Col Header in"=string[] ["지역", "구분", "설명"], "Data in"=w320) -> ("배열"=w318:string[], "Text out"=w317:string)  [unwired: 5 in, 2 out]
          n114 = Search 1D Array(1D array=w318, element=w317) -> (index of element=w315:i32)  [unwired: 1 in]
          n115 = Index Array(array=w316, index=w315) -> (element=w314:i32)
        }
      }
      n116 = Index Array(array=w285, index (row)=w286) -> (element=w288:string[])  [unwired: 1 in]
      n117 = Index Array(array=w288) -> (element #1=w296:string, element #2=w295:string)  [unwired: 2 in]
      n118 = Format Into String(format string="select A.TEMP, A.TTOL, A.HUMI, A.HTOL, B.DESN, A.ROOM_GUBUN, A.TIEM \nfrom autocal.TBLABMAN A, autocal.TBCALROM B \nwhere A.LOCT='%s'\nAND A.ROOM_GUBUN='%s'\nAND A.TIEM='%s'\nAND A.EMID='D-TECH' \nAND A.ROOM_GUBUN=B.ROOM_GUBUN", w296, w295, w291) -> (resulting string=w303:string)  [unwired: 2 in, 1 out]
    }
    frame "기관코드 얻기" {
      # "Get Basic Info"
      n119 = Unbundle By Name(w326) -> ("업체명"=w324:string)
      n120 = call <vilib>:"Trim Whitespace.vi"("string"=w324) -> ("trimmed string"=w322:string)  [unwired: 1 in]
      n121 = Format Into String(format string="select coid from autocal.tbsupman where conm='%s'", w322) -> (resulting string=w323:string)  [unwired: 2 in, 1 out]
    }
    frame "기술책임자 얻기" {
      # "Get Cal Director"
      n122 = Unbundle By Name(w335) -> ("문자열"=w328:string, "세부분류코드"=w331:string)
      n123 = Search and Replace String(input string=w331, search string="N0" ("검색 문자열")) -> (offset past replacement=w329:i32)  [unwired: 6 in, 3 out]
      n124 = case shown="-1" w329 {
        tunnel: ["select A.emid, B.emnm \nfrom autocal.tbcetman A, autocal.tbempman B\nwhere A.clas='기술책임자(정)' \nand A.emid=B.emid\nand A.calcod='%s' \nand not A.emid='T00215'" w345] -> w336
        tunnel: [w338 w344] -> w334
        tunnel: w331 -> [w339 w343]
        tunnel: w328 -> [_ w342]
        frame Default {
          n125 = String Subset(string=w339, offset (0)=2 ("오프셋(0)"), length (rest)=1 ("길이(나머지)")) -> (substring=w338:string)
        }
        frame -1 {
          n126 = case shown="\"02\"" w342 {
            tunnel: ["select A.emid, B.emnm \nfrom autocal.tbcetman A, autocal.tbempman B\nwhere A.clas='기술책임자(정)' \nand A.emid=B.emid\nand A.calcls='%s' \nand not A.emid='T00215'" "select A.emid, B.emnm \nfrom autocal.tbcetman A, autocal.tbempman B\nwhere A.clas='기술책임자(정)' \nand A.emid=B.emid\n%s\nand not A.emid='T00215'"] -> w345
            tunnel: [w348 " " ("세부분류코드")] -> w344
            tunnel: w343 -> [w346 _]
            frame Default {
              n127 = String Subset(string=w346, length (rest)=3 ("길이(나머지)")) -> (substring=w348:string)  [unwired: 1 in]
            }
            frame "02" {
            }
          }
        }
      }
      n128 = Format Into String(format string=w336, w334) -> (resulting string=w333:string)  [unwired: 2 in, 1 out]
    }
    frame "기준기등록리스트 얻기" {
      # "DB Manager"
      n129 = Unbundle By Name(w353) -> ("추가문자열"=w352:string)
      n130 = case shown="기본" w352 {
        selector: w352 -> [_ w359]
        tunnel: [_ w358] -> w356
        frame "" {
        }
        frame Default {
          n131 = Format Into String(format string="stdnam='%s' and " ("포맷 문자열"), w359) -> (resulting string=w358:string)  [unwired: 2 in, 1 out]
        }
      }
      n132 = Format Into String(format string="select distinct A.isid, C.conm, B.MODL, B.sern\nfrom TBCALSTD_MCT A, autocal.TBMASMAN B, autocal.TBSUPMAN C\nwhere %s\nA.isid=B.isid\nand B.mnfc=C.coid\norder by isid" ("SQL query"), w356) -> (resulting string=w354:string)  [unwired: 2 in, 1 out]
    }
    frame "기준기요청 얻기" {
      n133 = Unbundle By Name(w363) -> ("추가문자열"=w362:string, "등록번호"=w361:string)
      n134 = case shown="기본" w362 {
        tunnel: [w366 "select distinct \nA.isid, A.stdnam, C.conm, B.modl, A.caldate, A.regnam, SUBSTR(UPDATE_TIME,0, 10) \nfrom \ntbcalstd_mct_temp A, autocal.tbmasman B, autocal.tbsupman C \nwhere \nA.isid=B.isid \nand B.mnfc=C.coid \norder by stdnam, isid"] -> w364
        tunnel: w361 -> [w367 _]
        frame Default {
          n135 = Format Into String(format string="select * from tbcalstd_mct_temp where ISID='%s'", w367) -> (resulting string=w366:string)  [unwired: 2 in, 1 out]
        }
        frame "기준기요청리스트" {
        }
      }
    }
    frame "기책부책 얻기" {
    }
    frame "기타정보 얻기" {
      n136 = Unbundle By Name(w375) -> ("등록번호"=w372:string)
      n137 = Format Into String(format string="select\nA.part, A.mnfc, B.desn\nfrom\nautocal.tbmasman A, autocal.tbownpat B\nwhere isid='%s' and A.part=B.part", w372) -> (resulting string=w373:string)  [unwired: 2 in, 1 out]
    }
    frame "등록번호 얻기" {
      # "Get Registration Number"
      n138 = Unbundle By Name(w380) -> ("기기번호"=w379:string)
      n139 = Format Into String(format string="select A.isid, A.naem_sup, A.modl, B.conm, C.clsman, C.coddes\nfrom autocal.tbmasman A, autocal.tbsupman B, autocal.tbclsman C\nwhere A.sern='%s' \nand A.cust=B.coid\nand A.clsman_ext=C.clsman_ext\norder by A.naem, A.modl, A.isid, B.conm", w379) -> (resulting string=w378:string)  [unwired: 2 in, 1 out]
    }
    frame "등록정보 얻기" {
      # "Get Basic Info"
      n140 = Unbundle By Name(w384) -> ("등록번호"=w383:string)
      n141 = Format Into String(format string="select \nA.isid, B.conm, A.naem_sup, C.conm, A.modl, \nA.sern, A.clsman, A.clsman_ext, A.term, D.cidu, \nE.stdnam, E.calstd, D.kolas_mk, A.cust, F.desn, \nD.loct_pre, B.rpt_type, B.passht, A.mode_code, \nA.part, A.mnfc, G.desn, \nD.memo_cal, D.acc1, D.acc2, A.spc1 \nfrom\nautocal.tbmasman A, autocal.tbsupman B, autocal.tbsupman C, \nautocal.tbcalman D, autocal.tbclsman E, autocal.tbstaman F, \nautocal.tbownpat G \nwhere \nA.isid='%s'\nand A.cust=B.coid\nand A.mnfc=C.coid\nand A.clsman_ext=E.clsman_ext\nand A.isid=D.isid(+)\nand A.stat=F.stat\nand A.part=G.part\norder by casd desc, cidu desc" ("포맷 문자열"), w383) -> (resulting string=w382:string)  [unwired: 2 in, 1 out]
    }
    frame "모델(등록요청) 얻기" {
    }
    frame "모델(모델검색) 얻기" {
      n142 = Unbundle By Name(w392) -> ("세부분류코드"=w391:string, "형식"=w390:string, "옵션"=w389:string)
      n143 = case shown="기본" w389 {
        selector: w389 -> [w399 _]
        tunnel: [w398 _] -> w396
        frame Default {
          n144 = Format Into String(format string="and OPT_CODE like '%%%s%%'", w399) -> (resulting string=w398:string)  [unwired: 2 in, 1 out]
        }
        frame "" {
        }
      }
      n145 = case shown="기본" w391 {
        selector: w391 -> [w402 _]
        tunnel: [w401 _] -> w395
        frame Default {
          n146 = Format Into String(format string="CLSMAN_EXT='%s' and", w402) -> (resulting string=w401:string)  [unwired: 2 in, 1 out]
        }
        frame "ALL" {
        }
      }
      n147 = Format Into String(format string="select distinct CLSMAN_EXT, MDLMAN, OPT_CODE \nfrom TBCALPROC_MCT \nwhere %s \nMDLMAN like '%%%s%%' \n%s \norder by CLSMAN_EXT, MDLMAN, OPT_CODE", w395, w390, w396) -> (resulting string=w393:string)  [unwired: 2 in, 1 out]
    }
    frame "모델(범위조건) 얻기" {
      # "Start Create Procedure, Create Calibration Procedures"
      n148 = Unbundle By Name(w413) -> ("FUNC"=w411:string, "추가문자열"=w405:string, "FUNC_EXT"=w407:string, "옵션"=w409:string)
      n149 = case shown="기본" w407 {
        selector: w407 -> [w419 _]
        tunnel: [w418 _] -> w406
        frame Default {
          n150 = Format Into String(format string="AND FUNC_EXT='%s'", w419) -> (resulting string=w418:string)  [unwired: 2 in, 1 out]
        }
        frame "" {
        }
      }
      n151 = case shown="기본" w409 {
        selector: w409 -> [w422 _]
        tunnel: [w421 _] -> w408
        frame Default {
          n152 = Format Into String(format string="AND OPT_CODE='%s'", w422) -> (resulting string=w421:string)  [unwired: 2 in, 1 out]
        }
        frame "" {
        }
      }
      n153 = case shown="기본" w405 {
        selector: w405 -> [w417 _]
        tunnel: [w416 _] -> w404
        frame Default {
          n154 = Format Into String(format string="and c2_val ='%s'" ("포맷 문자열"), w417) -> (resulting string=w416:string)  [unwired: 2 in, 1 out]
        }
        frame "" {
        }
      }
      n155 = Format Into String(format string="select distinct mdlman, opt_code \nfrom tbcalproc_mct\nwhere\nfunc='%s'\n%s\n%s\n%s\norder by mdlman" ("SQL query"), w411, w404, w406, w408) -> (resulting string=w410:string)  [unwired: 2 in, 1 out]
    }
    frame "모델(조건별) 얻기" {
      n156 = Unbundle By Name(w428) -> ("세부분류코드"=w427:string, "항목명"=w425:string, "추가문자열"=w426:string)
      n157 = case shown="기본" w426 {
        selector: w426 -> [w435 _]
        tunnel: [w434 _] -> w424
        tunnel: w425 -> [w432 _]
        frame Default {
          n158 = Format Into String(format string="and %s ='%s'" ("포맷 문자열"), w432, w435) -> (resulting string=w434:string)  [unwired: 2 in, 1 out]
        }
        frame "" {
        }
      }
      n159 = Format Into String(format string="select DISTINCT \nMDLMAN, OPT_CODE, FUNC, FUNC_EXT, \nC1_VAL, C2_VAL, C3_VAL, C4_VAL, C5_VAL,\nC6_VAL, C7_VAL, C8_VAL, C9_VAL, C10_VAL \nfrom TBCALPROC_MCT\nwhere CLSMAN_EXT='%s'\n%s\nORDER BY MDLMAN, OPT_CODE", w427, w424) -> (resulting string=w429:string)  [unwired: 2 in, 1 out]
    }
    frame "모델(최대범위) 얻기" {
      # "Start Create Procedure"
      n160 = Unbundle By Name(w441) -> ("세부분류코드"=w436:string, "추가문자열"=w438:string)
      n161 = case shown="기본" w438 {
        selector: w438 -> [w445 _]
        tunnel: [w444 w448] -> w437
        tunnel: w436 -> [w443 w447]
        frame Default {
          n162 = Format Into String(format string="where clsman_ext='%s'\nand c2_val='%s'" ("포맷 문자열"), w443, w445) -> (resulting string=w444:string)  [unwired: 2 in, 1 out]
        }
        frame "" {
          n163 = Format Into String(format string="where clsman_ext='%s'" ("포맷 문자열"), w447) -> (resulting string=w448:string)  [unwired: 2 in, 1 out]
        }
      }
      n164 = Format Into String(format string="select distinct mdlman, opt_code \nfrom tbcalproc_mct \n%s\norder by mdlman" ("SQL query"), w437) -> (resulting string=w440:string)  [unwired: 2 in, 1 out]
    }
    frame "모델(최대최소) 얻기" {
      # "Start Create Procedure"
      n165 = Unbundle By Name(w456) -> ("세부분류코드"=w452:string, "배열 1"=w453:string[])
      n166 = Index Array(array=w453) -> (element #1=w451:string, element #2=w450:string)  [unwired: 2 in]
      n167 = Format Into String(format string="select distinct mdlman, opt_code \nfrom tbcalproc_mct \nwhere clsman_ext='%s'\nand c2_val='%s'\nand c3_val='%s'\norder by mdlman" ("SQL query"), w452, w451, w450) -> (resulting string=w455:string)  [unwired: 2 in, 1 out]
    }
    frame "모델(최소범위) 얻기" {
      # "Start Create Procedure"
      n168 = Unbundle By Name(w463) -> ("세부분류코드"=w458:string, "추가문자열"=w460:string)
      n169 = case shown="\"\"" w460 {
        selector: w460 -> [w467 _]
        tunnel: [w466 w470] -> w459
        tunnel: w458 -> [w465 w469]
        frame Default {
          n170 = Format Into String(format string="where clsman_ext='%s'\nand c3_val='%s'" ("포맷 문자열"), w465, w467) -> (resulting string=w466:string)  [unwired: 2 in, 1 out]
        }
        frame "" {
          n171 = Format Into String(format string="where clsman_ext='%s'" ("포맷 문자열"), w469) -> (resulting string=w470:string)  [unwired: 2 in, 1 out]
        }
      }
      n172 = Format Into String(format string="select distinct mdlman, opt_code \nfrom tbcalproc_mct \n%s\norder by mdlman" ("SQL query"), w459) -> (resulting string=w462:string)  [unwired: 2 in, 1 out]
    }
    frame "모델(항목전체) 얻기" {
      # "Start Create Procedure"
      n173 = Unbundle By Name(w475) -> ("세부분류코드"=w473:string)
      n174 = Format Into String(format string="select DISTINCT \nMDLMAN, OPT_CODE, FUNC, FUNC_EXT, \nC1_VAL, C2_VAL, C3_VAL, C4_VAL, C5_VAL,\nC6_VAL, C7_VAL, C8_VAL, C9_VAL, C10_VAL \nfrom TBCALPROC_MCT\nwhere CLSMAN_EXT='%s'\nORDER BY MDLMAN, OPT_CODE", w473) -> (resulting string=w472:string)  [unwired: 2 in, 1 out]
    }
    frame "모델(형식별) 얻기" {
      # "DB Manager"
      n175 = Unbundle By Name(w483) -> ("세부분류코드"=w480:string, "형식"=w479:string, "옵션"=w478:string)
      n176 = case shown="기본" w478 {
        selector: w478 -> [w486 _]
        tunnel: [w485 "AND OPT_CODE is null"] -> w477
        frame Default {
          n177 = Format Into String(format string="AND OPT_CODE='%s'", w486) -> (resulting string=w485:string)  [unwired: 2 in, 1 out]
        }
        frame "" {
        }
      }
      n178 = Format Into String(format string="select distinct MDLMAN, OPT_CODE \nFROM TBCALPROC_MCT\nwhere CLSMAN_EXT='%s'\nand MDLMAN='%s'\n%s", w480, w479, w477) -> (resulting string=w481:string)  [unwired: 2 in, 1 out]
    }
    frame "서버버전 얻기" {
    }
    frame "세부분류 목록 얻기" {
      # "DBM Initialize"
    }
    frame "업체정보 얻기" {
      # "Get Basic Info"
      n179 = Unbundle By Name(w495) -> ("업체명"=w494:string)
      n180 = Format Into String(format string="select \nrpt_type, passht \nfrom \nautocal.tbsupman \nwhere conm='%s'" ("포맷 문자열"), w494) -> (resulting string=w493:string)  [unwired: 2 in, 1 out]
    }
    frame "인증교정자 얻기" {
      # "Get Cal Manager"
      n181 = Unbundle By Name(w506) -> ("문자열"=w498:string, "사번"=w501:string, "세부분류코드"=w505:string)
      n182 = Search and Replace String(input string=w505, search string="N0" ("검색 문자열")) -> (offset past replacement=w499:i32)  [unwired: 6 in, 3 out]
      n183 = case shown="-1" w499 {
        tunnel: [w510 "select distinct A.emid, B.emnm \nfrom autocal.tbcetman A, autocal.tbempman B \nwhere not A.emid='%s' \nand not A.clas='기술책임자(정)' \nand not B.stat='퇴직자' \nand A.emid=B.emid \norder by emid"] -> w503
        tunnel: w505 -> [w511 _]
        tunnel: [w509 w518] -> w504
        tunnel: w501 -> [_ w518]
        tunnel: w498 -> [w508 _]
        frame -1 {
          n184 = case shown="기본" w508 {
            tunnel: w511 -> [w514 _]
            tunnel: ["select distinct A.emid, B.emnm \nfrom autocal.tbcetman A, autocal.tbempman B \nwhere A.calcls='%s' \nand not A.clas='기술책임자(정)' \nand not B.stat='퇴직자' \nand A.emid=B.emid \norder by emid" "select distinct A.emid, B.emnm \nfrom autocal.tbcetman A, autocal.tbempman B \nwhere %s \nnot A.clas='기술책임자(정)' \nand not B.stat='퇴직자' \nand A.emid=B.emid \norder by emid"] -> w510
            tunnel: [w512 " " ("세부분류코드")] -> w509
            frame Default {
              n185 = String Subset(string=w514, length (rest)=3 ("길이(나머지)")) -> (substring=w512:string)  [unwired: 1 in]
            }
            frame "02" {
            }
          }
        }
        frame Default {
        }
      }
      n186 = Format Into String(format string=w503, w504) -> (resulting string=w502:string)  [unwired: 2 in, 1 out]
    }
    frame "적용항목 얻기" {
    }
  }
  "Query" <- w3
  n187 = call "Get DB Data.vi"("error in (no error)"=w6, "SQL query"=w3, "connection reference"="참조 번호 입력") -> ("error out"=→"에러 출력":errorcluster, "Data"=w2:string[][], "connection reference"=→"참조 번호 출력":T3, "None?"=→"None?":bool)  [unwired: 4 in, 1 out]
  "Data" <- w2
  n188 = Index Array(array=w2) -> (element=→"Data (0번행)":string[])  [unwired: 2 in]
